vi "Select annot. for update.vi"(8 "error in":errorcluster, 10 "All cursors' dist.":T2) -> (0 "error out":errorcluster, 1 "Anott. for update":i32[](array[numeric]), 2 "All cursors' dist.":T2)   [LabVIEW 2014]
uses:
  Controls/dist. between cursors.ctl
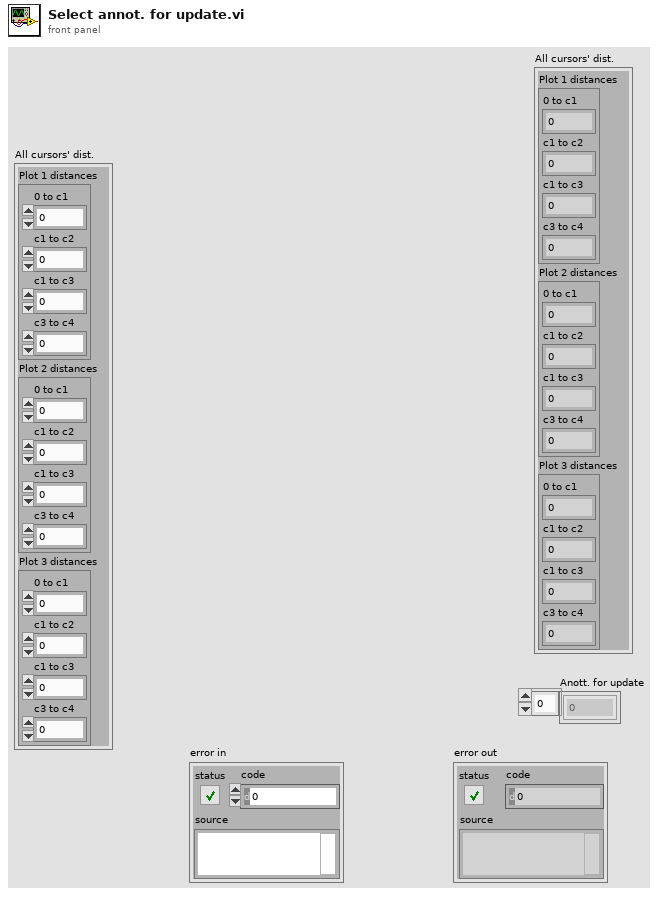
[diagram p1: front panel]
types:
  T1 = typedef "dist. between cursors.ctl" = cluster{"0 to c1":dbl, "c1 to c2":dbl, "c1 to c3":dbl, "c3 to c4":dbl}
  T2 = cluster{"Plot 1 distances":T1, "Plot 2 distances":T1, "Plot 3 distances":T1}
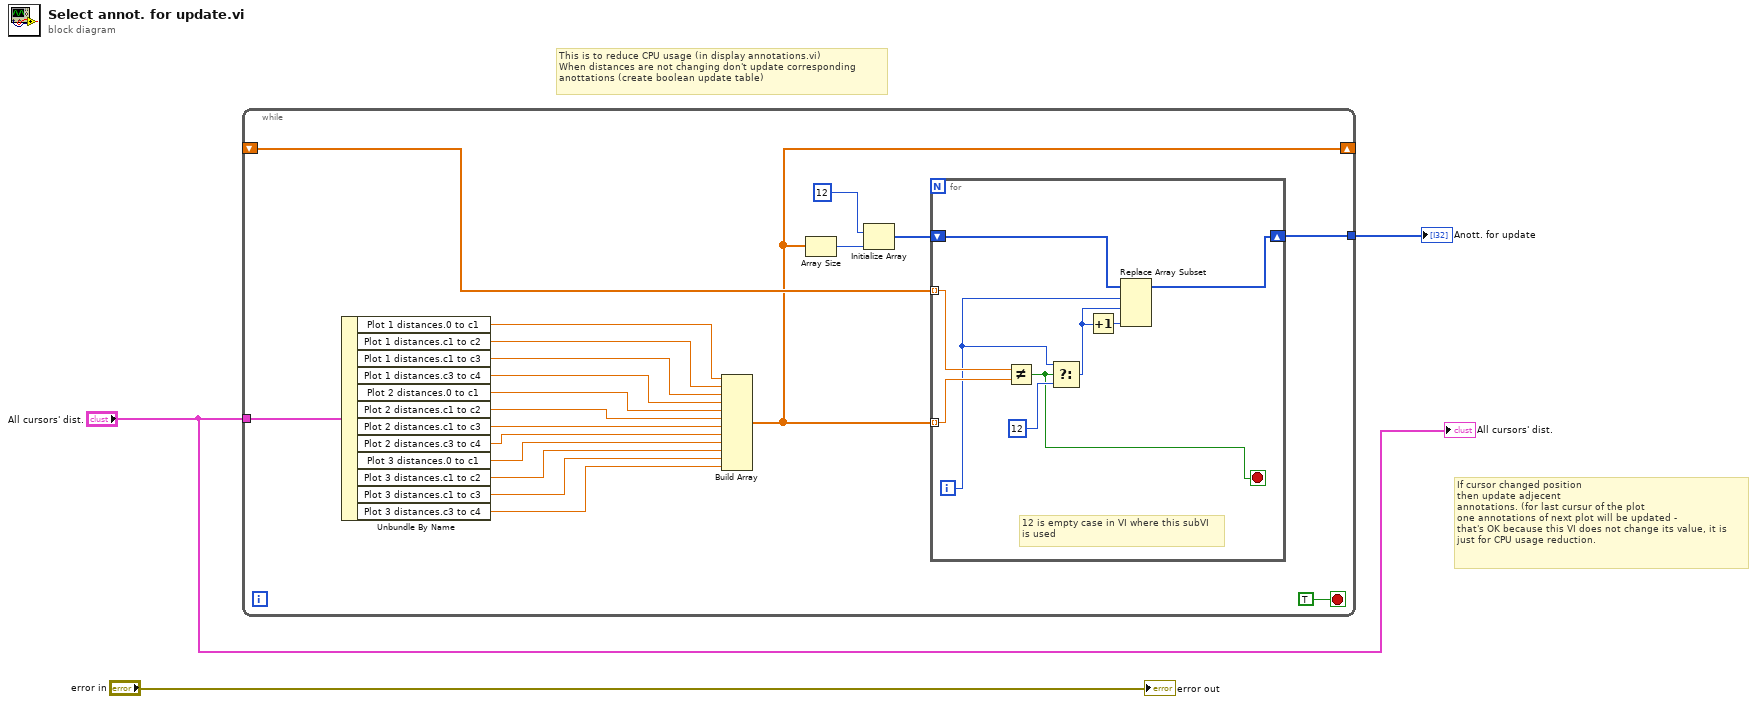
[diagram p0: block diagram]
diagram:
  # "If cursor changed position\nthen update adjecent \nannotations. (for last cursur of the plot \none annotations of next plot will be updated -\nthat's OK because this VI does not change its value, it is\njust for CPU usage reduction."
  # "This is to reduce CPU usage (in display annotations.vi)\nWhen distances are not changing don't update corresponding\nanottations (create boolean update table)"
  n1 = while {
    tunnel: "All cursors' dist." -> [w23]
    shift-right: [w6] -> _
    shift-left: _ -> [w7]
    tunnel: [w5] -> w2
    stop <- TRUE stop-if-true
    n2 = Unbundle By Name(w23) -> ("Plot 1 distances.0 to c1"=w11:dbl, "Plot 1 distances.c1 to c2"=w22:dbl, "Plot 1 distances.c1 to c3"=w21:dbl, "Plot 1 distances.c3 to c4"=w20:dbl, "Plot 2 distances.0 to c1"=w19:dbl, "Plot 2 distances.c1 to c2"=w18:dbl, "Plot 2 distances.c1 to c3"=w17:dbl, "Plot 2 distances.c3 to c4"=w16:dbl, "Plot 3 distances.0 to c1"=w15:dbl, "Plot 3 distances.c1 to c2"=w14:dbl, "Plot 3 distances.c1 to c3"=w13:dbl, "Plot 3 distances.c3 to c4"=w12:dbl)
    n3 = Build Array(w11, w22, w21, w20, w19, w18, w17, w16, w15, w14, w13, w12) -> (w6:dbl[])
    n4 = Array Size(array=w6) -> (size(s)=w10:i32)
    n5 = Initialize Array(12, w10) -> (w9:i32[])
    n6 = for {
      tunnel: w6 -> [w31] mode=indexing
      tunnel: w7 -> [w32] mode=indexing
      shift-right: [w29] -> w5
      shift-left: w9 -> [w30]
      i -> [w24]
      stop <- w27 stop-if-true
      # "12 is empty case in VI where this subVI\nis used"
      n7 = Not Equal?(x=w32, y=w31) -> (x != y?=w27:bool)
      n8 = Select(t=w24, s=w27, f=12) -> (s? t:f=w26:i32)
      n9 = Increment(x=w26) -> (x+1=w25:i32)
      n10 = Replace Array Subset "Replace Array Subset"(array=w30, new element #1=w26, index #1=w24, new element #2=w25) -> (w29:i32[])  [unwired: 1 in]
    }
  }
  "Anott. for update" <- w2
  "error out" <- "error in"
  "All cursors' dist." <- "All cursors' dist."
